vi "dynanometer_DAQ_digital_output _line0_1.vi"() -> ()   [LabVIEW 2015]
uses:
  <vilib>/Vernier/SensorDAQ/Low Level Drivers/SensorDAQ Controls/Config Ch 1-3 Enum.ctl
  <vilib>/Vernier/SensorDAQ/Low Level Drivers/SensorDAQ Controls/Collection Parameters Enum.ctl
  <vilib>/Utility/file.llb/Write Delimited Spreadsheet (DBL).vi
panel:
  in  "Save to File":bool=TRUE
  in  "Threshold for Ch. 2 (N)":dbl=10.0
  out "Comparison for Ch. 2":bool[](array[boolean])
  out "Comparison for Ch. 1":bool[](array[boolean])
  in  "Threshold for Ch. 1 (N)":dbl=10.0
  out "Ch. 2 Chart":dbl[](graph)
  out "Total # of samples":i32
  out "Time per sample \n(s/sample)":dbl
  out "AI1 Chart":dbl[](graph)
  out "AI0 Chart":dbl[](graph)
  out "Ch. 1 Chart":dbl[](graph)
  in  "?":bool
  out "SensorDAQ Connected?":bool
  in  "AI1 Configuration":T1(ring)=enum."AI1 0-5V RSE"
  in  "AI0 Configuration":T2(ring)=enum."AI0 0-5V RSE"
  in  "Repeat Collection?":bool
  in  "Samples to be Collected":dbl=20000.0
  in  "Sampling Rate (samples/s)":dbl=20.0
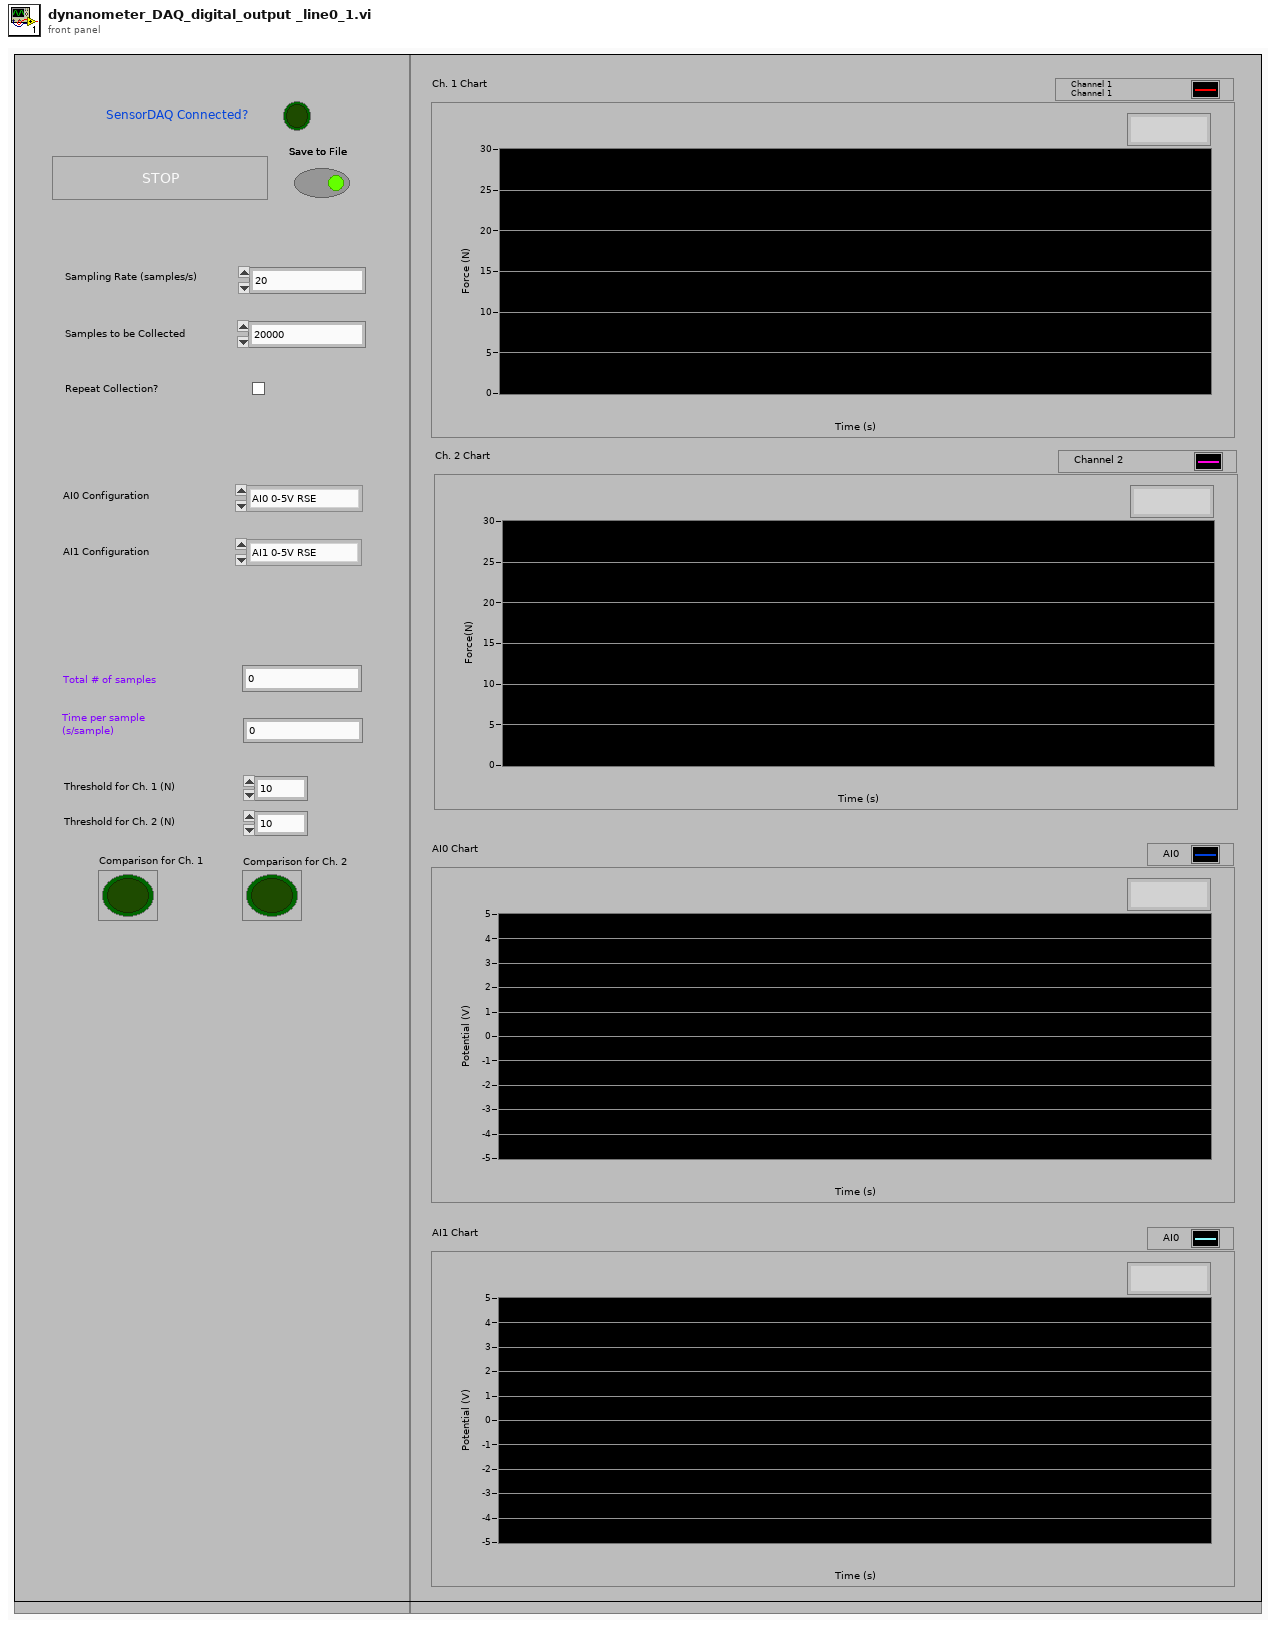
[diagram p1: front panel]
types:
  T1 = enum16{"AI1 OFF", "AI1 0-5V RSE", "AI1 +-10V RSE"}
  T2 = enum16{"AI0 OFF", "AI0 0-5V RSE", "AI0 +-10V RSE", "AI0 Differential"}
  T3 = typedef "Collection Parameters Enum.ctl" = enum16{"Modify with Inputs into this subVI", "Modify with Data Collection Popup ", "Modify with Calibration File Popup", "Modify with Select Units Popup", "Modify with Zero Reading Popup", "Get Current Parameters", "Init", "In Probe Data", "In New Parameters"}
  T4 = typedef "Config Ch 1-3 Enum.ctl" = enum16{"OFF", "ON ", "ON - Use \"Custom Ch\" Input Values"}
  T5 = typedef "DAQmx Task Cluster.ctl" = cluster{"DIG Ch Task":refnum<k21>, "P0<0:3> DigOut Task":refnum<k21>, "P0<0:3> DigIn Task":refnum<k21>, "AO 0 Task":refnum<k21>, "PFI 0 Task":refnum<k21>, "Ch1-3 AI0 AI1 Task":refnum<k21>, "SensorDAQ Device":tag}
  T6 = typedef "Setup Parameters Cluster.ctl" = cluster{"Config Ch1-3, AI0, AI1":T7, "Config DIG Ch":T11, "Config DIO":T13, "Config AO":T15, "Config Counter":T16}
  T7 = typedef "Config Ch1-3, AI0, AI1 Cluster.ctl" = cluster{"Sensor Info Array":T8[], "CH1 Y min":dbl, "CH2 Y min":dbl, "CH3 Y min":dbl, "AI0 Y min":dbl, "AI1 Y min":dbl, "CH1 Y max":dbl, "CH2 Y max":dbl, "CH3 Y max":dbl, "AI0 Y max":dbl, "AI1 Y max":dbl, "X min":dbl, "X max":dbl, "sample rate (sample/sec)":dbl, "sample time (sec/sample)":dbl, "# of samples":u32, "Repeat?":bool, "Active Channel Array":bool[], "# active probes":u32, "TrigType":T9, "TrigChan":i32, "TrigThresh":dbl, "Pre-Store (%)":i32, "Pre-store (#samp)":u32, "Short Sensor Name":string[], "Product ID Array":u8[], "AI0 Configuration":enum16{"AI0 OFF", "AI0 0-5V RSE", "AI0 +-10V RSE", "AI0 Differential"}, "AI1 Configuration":enum16{"AI1 OFF", "AI1 0-5V RSE", "AI1 +-10V RSE"}, "Averaging Enum":T10}
  T8 = typedef "Sensor Info Cluster.ctl" = cluster{"Long Name":string, "Active CalPage":u8, "Calpage Coefficients":cluster{"K0":sgl, "K1":sgl, "K2":sgl, "Units":string}[], "Equation Type":u8, "Operation Type":u8, "Num Valid Cal Pages":u8}
  T9 = typedef "TrigType Enum.ctl" = enum16{"No Trigger", "DIG Channel Trigger - Rising Edge", "DIG Channel Trigger - Falling Edge", "Screw Terminal (PFI.0) - Rising Edge", "Screw Terminal (PFI.0) - Falling Edge", "Analog Trigger - Threshold Above", "Analog Trigger - Threshold Below", "Analog Trigger - Rising", "Analog Trigger - Falling"}
  T10 = typedef "Averaging Enum.ctl" = enum16{"Averaging On", "Averaging Off"}
  T11 = typedef "Config DIG Channel Cluster.ctl" = cluster{"Config DIG Channel (OFF)":T12, "sample rate\n(sample/sec)":dbl, "# of samples":u32, "Y min":dbl, "Y max":dbl, "X min":dbl, "X max":dbl}
  T12 = typedef "Config DIG Channel Enum.ctl" = enum16{"OFF", "Photogate Simple Counting", "Photogate Single Timed Count", "Photogate Timing (Semi-Period)", "Photogate Timing (Period)", "Photogate Timing (2 Edge)", "Motion Detector", "DCU", "DCU - Pulse Train (line D1)", "Rotary Motion Sensor", "Radiation Monitor", "Heat Pulser"}
  T13 = typedef "Config DI0 Terminals Cluster.ctl" = cluster{"Dig Line P0.0":T14, "Dig Line P0.1":T14, "Dig Line P0.2":T14, "Dig Line P0.3":T14}
  T14 = typedef "Config DIO Line Enum.ctl" = enum16{"OFF", "ON - Digital In", "ON - Digital Out"}
  T15 = typedef "Config Analog Out Enum.ctl" = enum16{"OFF", "ON"}
  T16 = typedef "Config Counter Enum.ctl" = enum16{"OFF", "Simple Edge Counting", "Semi-Period Measurement", "Period Measurement", "Two Edge Separation", "Pulse Train Generation"}
  T17 = typedef "NI_Matrix.lvlib/RealMatrix.ctl" = dbl[][]
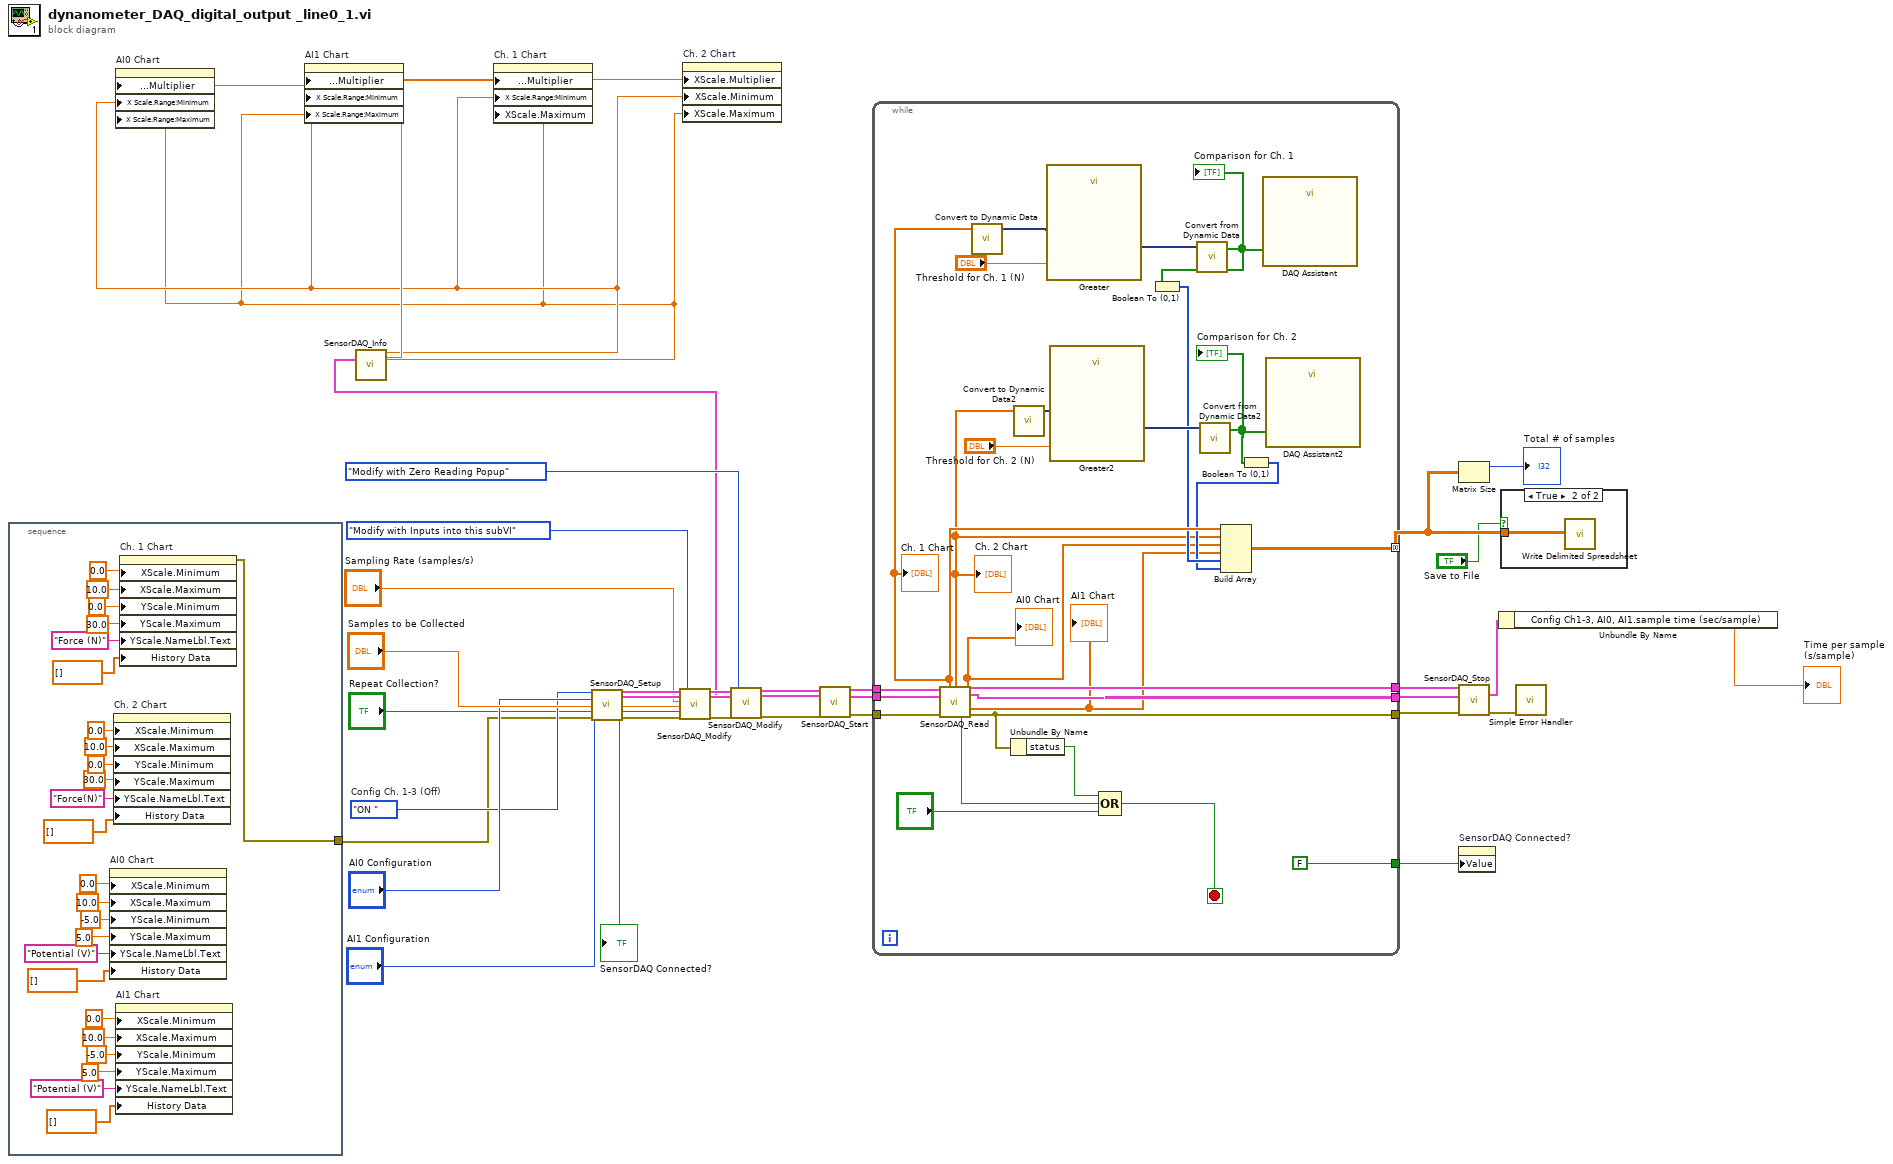
[diagram p0: block diagram]
diagram:
  w31 = Config_Ch_1-3_Enum."ON "  # Config Ch. 1-3 (Off)
  n1 = stacked-sequence {
    tunnel: [w42] -> w11
    frame #0 {
      n2 = property on="AI0 Chart" class="WFChart (strict)"("XScale.Minimum"=0.0, "XScale.Maximum"=10.0, "YScale.Minimum"=-5.0, "YScale.Maximum"=5.0, "YScale.NameLbl.Text"="Potential (V)", "History Data"=dbl[] [] ("Ch. 1 Graph")) -> ()  [unwired: 2 in, 2 out]
      n3 = property on="Ch. 2 Chart" class="WFChart (strict)"("XScale.Minimum"=0.0 ("X Scale.Range:Minimum"), "XScale.Maximum"=10.0 ("X Scale.Range:Maximum"), "YScale.Minimum"=0.0 ("Y Scale.Range:Minimum"), "YScale.Maximum"=30.0 ("Y Scale.Range:Maximum"), "YScale.NameLbl.Text"="Force(N)" ("Y Scale.Name Label.Text"), "History Data"=dbl[] []) -> ()  [unwired: 2 in, 2 out]
      n4 = property on="AI1 Chart" class="WFChart (strict)"("XScale.Minimum"=0.0, "XScale.Maximum"=10.0, "YScale.Minimum"=-5.0, "YScale.Maximum"=5.0, "YScale.NameLbl.Text"="Potential (V)", "History Data"=dbl[] [] ("Ch. 1 Graph")) -> ()  [unwired: 2 in, 2 out]
      n5 = property on="Ch. 1 Chart" class="WFChart (strict)"("XScale.Minimum"=0.0, "XScale.Maximum"=10.0, "YScale.Minimum"=0.0, "YScale.Maximum"=30.0, "YScale.NameLbl.Text"="Force (N)", "History Data"=dbl[] [] ("Ch. 1 Graph")) -> (error out=w42:errorcluster)  [unwired: 2 in, 1 out]
    }
  }
  n6 = call <vilib>:"SensorDAQ_Setup.vi"("Config Ch. 1-3 (Off)"=w31, "AI0 Configuration (Off)"="AI0 Configuration", "AI1 Configuration (Off)"="AI1 Configuration", "error in (no error)"=w11) -> ("DAQmx Task Cluster"=w35:T5, "Setup Parameters"=w34:T6, "SensorDAQ Connected?"=→"SensorDAQ Connected?":bool, "Error Out"=w24:errorcluster)  [unwired: 8 in]
  n7 = call <vilib>:"SensorDAQ_Modify.vi"("DAQmx Task Cluster"=w35, "Setup Parameters"=w34, "Sample Rate (samples/sec)"="Sampling Rate (samples/s)", "Samples to be Collected"="Samples to be Collected", "Repeat Collection?"="Repeat Collection?", "error in (no error)"=w24, "Collection Parameters Enum"=Collection_Parameters_Enum."Modify with Inputs into this subVI") -> ("DAQmx Task Cluster out"=w21:T5, "Setup Parameters"=w20:T6, "error out"=w16:errorcluster)  [unwired: 8 in, 2 out]
  n8 = call <vilib>:"SensorDAQ_Modify.vi"("DAQmx Task Cluster"=w21, "Setup Parameters"=w20, "error in (no error)"=w16, "Collection Parameters Enum"=Collection_Parameters_Enum."Modify with Zero Reading Popup") -> ("DAQmx Task Cluster out"=w17:T5, "Setup Parameters"=w4:T6, "error out"=w15:errorcluster)  [unwired: 11 in, 2 out]
  n9 = call <vilib>:"SensorDAQ_Info.vi"("Setup Parameters"=w4) -> ("X Multiplier"=w10:dbl, "X min"=w9:dbl, "X max"=w8:dbl)  [unwired: 7 in, 5 out]
  n10 = property on="AI0 Chart" class="WFChart (strict)"("X Scale.Offset and Multiplier:Multiplier"=w10, "X Scale.Range:Minimum"=w9, "X Scale.Range:Maximum"=w8) -> ()  [unwired: 2 in, 2 out]
  n11 = property on="AI1 Chart" class="WFChart (strict)"("X Scale.Offset and Multiplier:Multiplier"=w10, "X Scale.Range:Minimum"=w9, "X Scale.Range:Maximum"=w8) -> ()  [unwired: 2 in, 2 out]
  n12 = property on="Ch. 1 Chart" class="WFChart (strict)"("X Scale.Offset and Multiplier:Multiplier"=w10, "X Scale.Range:Minimum"=w9, "XScale.Maximum"=w8) -> ()  [unwired: 2 in, 2 out]
  n13 = property on="Ch. 2 Chart" class="WFChart (strict)"("XScale.Multiplier"=w10, "XScale.Minimum"=w9, "XScale.Maximum"=w8) -> ()  [unwired: 2 in, 2 out]
  n14 = call <vilib>:"SensorDAQ_Start.vi"("DAQmx Task Cluster"=w17, "Setup Parameters"=w4, "error in"=w15) -> ("DAQmx Task Cluster out"=w28:T5, "Setup Parameters"=w27:T6, "error out"=w26:errorcluster)  [unwired: 10 in]
  n15 = while {
    tunnel: w28 -> [w76]
    tunnel: w27 -> [w75]
    tunnel: w26 -> [w77]
    tunnel: [w86] -> w5
    tunnel: [w85] -> w25
    tunnel: [w84] -> w6
    tunnel: [FALSE] -> w23
    tunnel: [w78] -> w3 mode=concatenating
    stop <- w83 stop-if-true
    n16 = call <vilib>:"SensorDAQ_Read.vi"("DAQmx Task Cluster"=w76, "Setup Parameters"=w75, "error in"=w77) -> ("CH 1"=w73:dbl[], "CH 2"=w63:dbl[], "DAQmx Task Cluster"=w86:T5, "Setup Parameters"=w85:T6, "AI0"=w61:dbl[], "AI1"=w62:dbl[], "Collection Done"=w80:bool, "error out"=w84:errorcluster)  [unwired: 2 in, 3 out]
    "Ch. 1 Chart" <- w73
    "AI0 Chart" <- w61
    "AI1 Chart" <- w62
    "Ch. 2 Chart" <- w63
    n17 = call "Convert to Dynamic Data"("Array"=w73) -> ("Dynamic Data Type"=w72:dynamicdata)  [unwired: 3 in]
    n18 = Unbundle By Name(w84) -> ("status"=w82:bool)
    n19 = call "Convert to Dynamic Data2"("Array"=w63) -> ("Dynamic Data Type"=w70:dynamicdata)  [unwired: 3 in]
    n20 = call "Greater"("Operand 2"="Threshold for Ch. 1 (N)", "Operand 1"=w72) -> ("Result"=w74:dynamicdata)  [unwired: 8 in, 1 out]
    n21 = call "Greater2"("Operand 2"="Threshold for Ch. 2 (N)", "Operand 1"=w70) -> ("Result"=w71:dynamicdata)  [unwired: 8 in, 1 out]
    n22 = Compound Arithmetic op=OR(w82, w80, "?") -> (w83:bool)
    n23 = call "Convert from Dynamic Data"("Dynamic Data Type"=w74) -> ("Array"=w67:bool[])  [unwired: 3 in]
    "Comparison for Ch. 1" <- w67
    n24 = Boolean To (0,1)(Boolean=w67) -> (0, 1=w66:i16[])
    n25 = call "Convert from Dynamic Data2"("Dynamic Data Type"=w71) -> ("Array"=w65:bool[])  [unwired: 3 in]
    "Comparison for Ch. 2" <- w65
    n26 = Boolean To (0,1)(Boolean=w65) -> (0, 1=w64:i16[])
    n27 = Build Array(w73, w63, w61, w62, w66, w64) -> (w78:T17)
    n28 = call "DAQ Assistant"("data"=w67) -> ()  [unwired: 17 in, 2 out]
    n29 = call "DAQ Assistant2"("data"=w65) -> ()  [unwired: 17 in, 2 out]
  }
  n30 = Matrix Size(0:w3) -> (1:→"Total # of samples":i32)  [unwired: 1 out]
  n31 = call <vilib>:"SensorDAQ_Stop.vi"("DAQmx Task Cluster"=w5, "Setup Parameters"=w25, "error in"=w6) -> ("Setup Parameters"=w14:T6, "error out"=w7:errorcluster)  [unwired: 10 in, 1 out]
  n32 = property on="SensorDAQ Connected?" class="Bool (strict)"("Value"=w23) -> ()  [unwired: 2 in, 2 out]
  n33 = Unbundle By Name(w14) -> ("Config Ch1-3, AI0, AI1.sample time (sec/sample)"=→"Time per sample \n(s/sample)":dbl)
  n34 = case shown="True" "Save to File" {
    tunnel: w3 -> [_ w87]
    frame False {
    }
    frame True {
      n35 = call-poly <vilib>:"Write Delimited Spreadsheet.vi"("2D data"=w87) -> ()  [unwired: 13 in, 2 out]
    }
  }
  n36 = call <vilib>:"Simple Error Handler.vi"("error in (no error)"=w7) -> ()  [unwired: 4 in, 5 out]
